vi "DAQmx Create Channel (CI-Period).vi"(0 "task in":refnum<k21>, 1 "maximum value":dbl=0.1 format="%0.6f", 2 "minimum value":dbl=1e-06 format="%0.6f", 3 "measurement method":i32(ring)=10105 items=["Low Frequency with 1 Counter"=10105, "High Frequency with 2 Counters"=10157, "Large Range with 2 Counters"=10205, "Dynamic Averaging"=16065], 5 "counter":tag, 6 "divisor":u32=4, 7 "name to assign":string, 9 "units":i32(ring)=10364 items=["Seconds"=10364, "Ticks"=10304, "From Custom Scale"=10065], 11 "error in":errorcluster, 12 "custom scale name":tag, 13 "starting edge":i32(ring)=10280 items=["Rising"=10280, "Falling"=10171], 14 "measurement time":dbl=0.001 format="%0.6f") -> (4 "task out":refnum<k21>, 15 "error out":errorcluster)   [LabVIEW 2013]
doc: "Creates a channel to measure the period of a digital signal. With the exception of devices that support multi-counter tasks, you can create only one counter input channel at a time with this VI because a task can contain only one counter input channel. To read from multiple counters simultaneously, use a separate task for each counter. Connect the input signal to the default input terminal of the counter unless you select a different input terminal."
uses:
  <resource>/objmgr/daqmx.rc
panel:
  # "input limits"
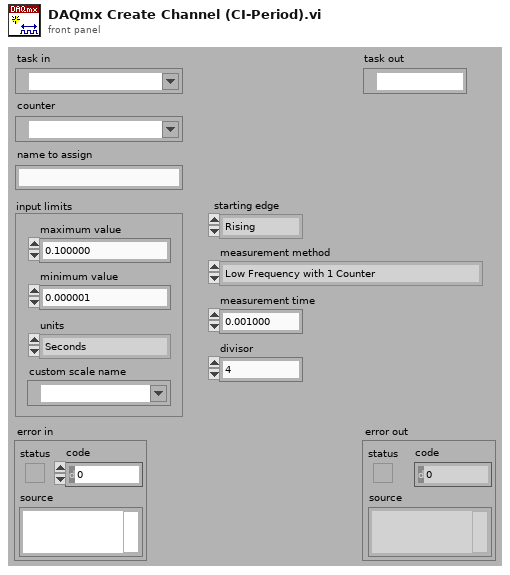
[diagram p1: front panel]
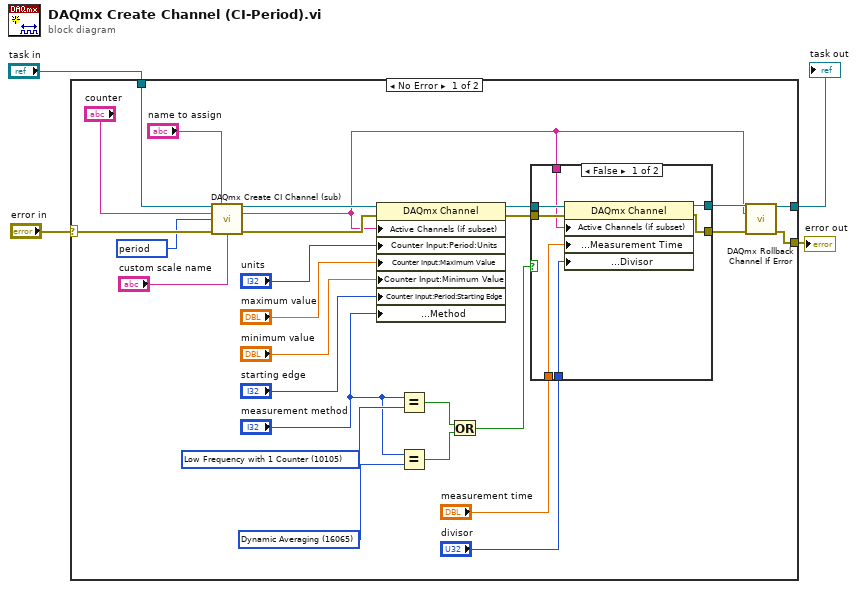
[diagram p0: block diagram]
diagram:
  n1 = case shown="No Error" "error in" {
    selector: "error in" -> [w30 w41]
    tunnel: "task in" -> [w31 w42]
    tunnel: [w19 w42] -> w2
    tunnel: [w18 w41] -> w1
    frame No Error {
      w9 = 16065 items=["Low Frequency with 1 Counter"=10105, "High Frequency with 2 Counters"=10157, "Large Range with 2 Counters"=10205, "Dynamic Averaging"=16065] ("CI.Period.MeasMeth")
      w11 = 10105 items=["Low Frequency with 1 Counter"=10105, "High Frequency with 2 Counters"=10157, "Large Range with 2 Counters"=10205, "Dynamic Averaging"=16065] ("CI.Period.MeasMeth")
      w24 = 10256 items=["count events"=10125, "frequency"=10179, "period"=10256, "pulse width"=10267, "semi period"=10289] ("measurement type")
      n2 = call "DAQmx Create CI Channel (sub).vi"("task in"=w31, "virtual channel name"="name to assign", "physical channel name"="counter", "measurement type"=w24, "error in"=w30, "custom scale"="custom scale name") -> ("task out"=w20:refnum<k21>, "channel names"=w5:string, "error out"=w28:errorcluster)  [unwired: 7 out]
      n3 = property class="DAQmx Channel"(reference=w20, error in=w28, "Active Channels (if subset)"=w5, "Counter Input:Period:Units"="units", "Counter Input:Maximum Value"="maximum value", "Counter Input:Minimum Value"="minimum value", "Counter Input:Period:Starting Edge"="starting edge", "Counter Input:Period:Measurement Specifications:Method"="measurement method") -> (reference out=w17:refnum<k21>, error out=w16:errorcluster)
      n4 = Equal?(x="measurement method", y=w11) -> (x = y?=w8:bool)
      n5 = Equal?(x="measurement method", y=w9) -> (x = y?=w7:bool)
      n6 = Or(x=w8, y=w7) -> (x .or. y?=w6:bool)
      n7 = case shown="False" w6 {
        tunnel: w17 -> [w38 w40]
        tunnel: w16 -> [w37 w39]
        tunnel: [w36 w40] -> w15
        tunnel: [w35 w39] -> w14
        tunnel: "measurement time" -> [w34 _]
        tunnel: "divisor" -> [w33 _]
        tunnel: w5 -> [w32 _]
        frame False {
          n8 = property class="DAQmx Channel"(reference=w38, error in=w37, "Active Channels (if subset)"=w32, "Counter Input:Period:Measurement Specifications:High Frequency:Measurement Time"=w34, "Counter Input:Period:Measurement Specifications:Large Range:Divisor"=w33) -> (reference out=w36:refnum<k21>, error out=w35:errorcluster)
        }
        frame True {
        }
      }
      n9 = call "DAQmx Rollback Channel If Error.vi"("task in"=w15, "channel names"=w5, "error in"=w14) -> ("task out"=w19:refnum<k21>, "error out"=w18:errorcluster)  [unwired: 11 out]
    }
    frame Error {
    }
  }
  "error out" <- w1
  "task out" <- w2
